vi "CSM - Remove Duplicated Following Messages.vi"(2 "Current State":string, 3 "Remaining States":string) -> (1 "Remaining States Left":string)   [LabVIEW 2020, in "Communicable State Machine.lvlib"]
uses:
  Communicable State Machine.lvlib
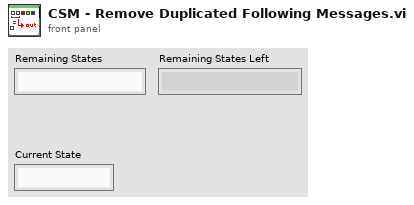
[diagram p1: front panel]
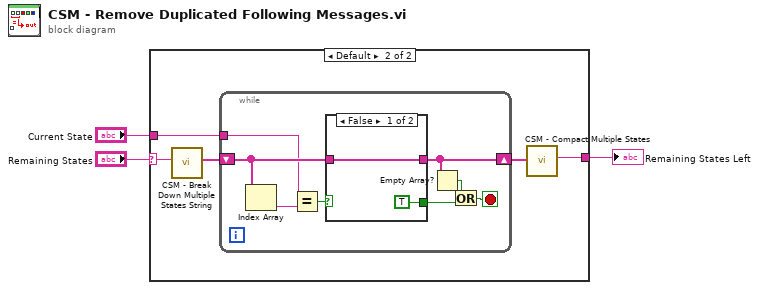
[diagram p0: block diagram]
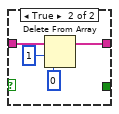
[diagram p3: hidden frame]
diagram:
  n1 = case shown="Default" "Remaining States" {
    selector: "Remaining States" -> [w4 w5]
    tunnel: [w4 w9] -> w3
    tunnel: "Current State" -> [_ w7]
    frame "" {
    }
    frame Default {
      n2 = call "CSM - Break Down Multiple States String.vi"("States"=w5) -> ("Multiple States"=w6:string[])  [unwired: 10 in]
      n3 = while {
        tunnel: w7 -> [w15]
        shift-right: [w13] -> w8
        shift-left: w6 -> [w17]
        stop <- w12 stop-if-true
        n4 = Index Array(array=w17) -> (element=w16:string)  [unwired: 1 in]
        n5 = Equal?(x=w15, y=w16) -> (x = y?=w14:bool)
        n6 = case shown="False" w14 {
          tunnel: w17 -> [w19 w23]
          tunnel: [w19 w22] -> w13
          tunnel: [TRUE _] -> w11
          frame False {
          }
          frame True {
            n7 = Delete From Array(array=w23, length=1, index=0) -> (array with subset deleted=w22:string[])  [unwired: 1 out]
          }
        }
        n8 = Empty Array?(array=w13) -> (empty?=w10:bool)
        n9 = Or(x=w10, y=w11) -> (x .or. y?=w12:bool)
      }
      n10 = call "CSM - Compact Multiple States.vi"("Multiple States"=w8) -> ("States"=w9:string)  [unwired: 9 in]
    }
  }
  "Remaining States Left" <- w3
